vi "Add class.vi"(8 "Error In":errorcluster, 10 "Class label":string, 11 "Ctl path":path) -> (0 "Error Out":errorcluster)   [LabVIEW 2016]
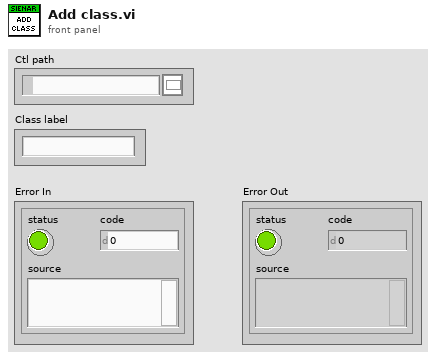
[diagram p1: front panel]
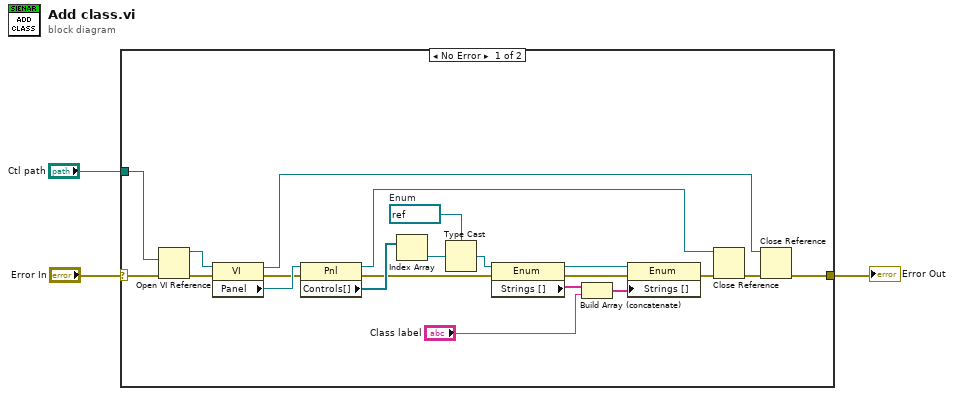
[diagram p0: block diagram]
diagram:
  n1 = case shown="No Error" "Error In" {
    selector: "Error In" -> [w4 w25]
    tunnel: "Ctl path" -> [w6 _]
    tunnel: [w5 w25] -> w2
    frame No Error {
      w20 = refnum<vi> refnum  # Enum
      n2 = Open VI Reference(vi path=w6, error in (no error)=w4) -> (vi reference=w24:refnum<vi>, error out=w8:errorcluster)  [unwired: 4 in]
      n3 = property class="VI"(reference=w24, error in=w8) -> (reference out=w19:refnum<vi>, error out=w17:errorcluster, "Panel"=w23:refnum<vi>)
      n4 = property class="Pnl"(reference=w23, error in=w17) -> (reference out=w18:refnum<vi>, error out=w16:errorcluster, "Controls[]"=w22:refnum<vi>[])
      n5 = Index Array(array=w22) -> (element=w21:refnum<vi>)  [unwired: 1 in]
      n6 = Type Cast(type=w20, x=w21) -> (*(type *) &x=w9:refnum<vi>)
      n7 = property class="Enum"(reference=w9, error in=w16) -> (reference out=w14:refnum<vi>, error out=w11:errorcluster, "Strings []"=w13:string[])
      n8 = Build Array (concatenate)(w13, "Class label") -> (w12:string[])
      n9 = property class="Enum"(reference=w14, error in=w11, "Strings []"=w12) -> (error out=w10:errorcluster)  [unwired: 1 out]
      n10 = Close Reference(reference=w18, error in (no error)=w10) -> (error out=w15:errorcluster)
      n11 = Close Reference(reference=w19, error in (no error)=w15) -> (error out=w5:errorcluster)
    }
    frame Error {
    }
  }
  "Error Out" <- w2
